vi "create data log.vi"(0 "Header String":string="This is a log file of a temperature control run being done in Physics 3600 for the bug experiment. It records the time, temperature, power, and control setting for each PID update. It does so by accumulating the data and periodically saving it.", 11 "PID exp exec in":T1) -> (4 "exists":bool=TRUE, 15 "PID exp exec out":T1)   [LabVIEW 2019]
doc: "This vi prompts the user to choose whether to create a data log. If the user so chooses, a temp parameters log file is created with the given header.\n\nPaul K Dixon\nPhysics 3600\nCSUSB Physics"
uses:
  typedefs/PID exec cluster.ctl
  typedefs/bug temp file info.ctl
  globals/Bug temp globals.vi
panel:
  out "temp log file path":path
  in  "String":string="Time (ms)\tTemp (C)\tPower\tSetpoint\tCB\tItime\tIon\tDtime\tDon\tSB\tStime\tTime in SB\tSettled\tMan Pow\tMan on"
  out "file refnum out":refnum<file>
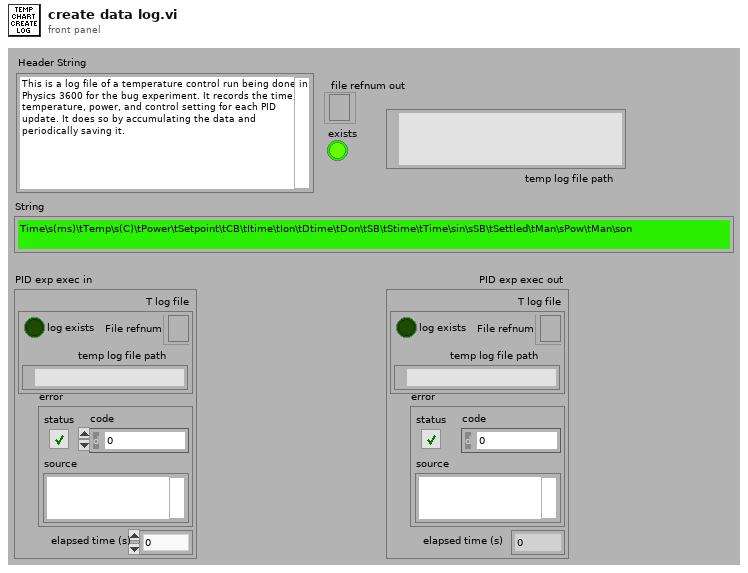
[diagram p1: front panel]
types:
  T1 = typedef "PID exec cluster.ctl" = cluster{"T log file":T2, "error":errorcluster, "elapsed time (s)":dbl}
  T2 = typedef "bug temp file info.ctl" = cluster{"log exists":bool, "File refnum":refnum<file>, "temp log file path":path}
  T3 = typedef "temp cont cluster.ctl" = cluster{"exec":T4, "T status":T6, "T params":T8, "utility":T9}
  T4 = typedef "temp exec cluster.ctl" = cluster{"T mode":T5, "exec setpoint":dbl, "reset":bool, "man power":dbl, "man":bool, "log":bool, "clear":bool}
  T5 = typedef "temp mode enum.ctl" = enum16{"Setting up", "Listening to exec", "Exit"}
  T6 = typedef "temp indicator.ctl" = cluster{"Control status":T7, "Temp":dbl, "Power":dbl, "Time in settle band":dbl, "Settled":bool, "Low":bool, "High":bool, "Setpoint":dbl, "Control":bool, "In Settle Band":bool}
  T7 = typedef "temp control status.ctl" = enum16{"In Settle Band", "In Control Band", "Below Control Band", "Above Control Band"}
  T8 = typedef "PID control parameters.ctl" = cluster{"Setpoint":dbl, "Control Bandwidth":dbl, "Integral Time":dbl, "Int\nON":bool, "Derivative Tme":dbl, "Der\nON":bool, "Settle Bandwidth":dbl, "Settle Time":dbl}
  T9 = typedef "temp cont utility.ctl" = cluster{"meas index":i32, "wait (ms)":i32, "H Vmax":dbl, "power out":dbl, "heat volt out":dbl, "heat volt in":dbl, "therm volt":dbl, "t T P hist":dbl[][], "cont hist":dbl[][]}
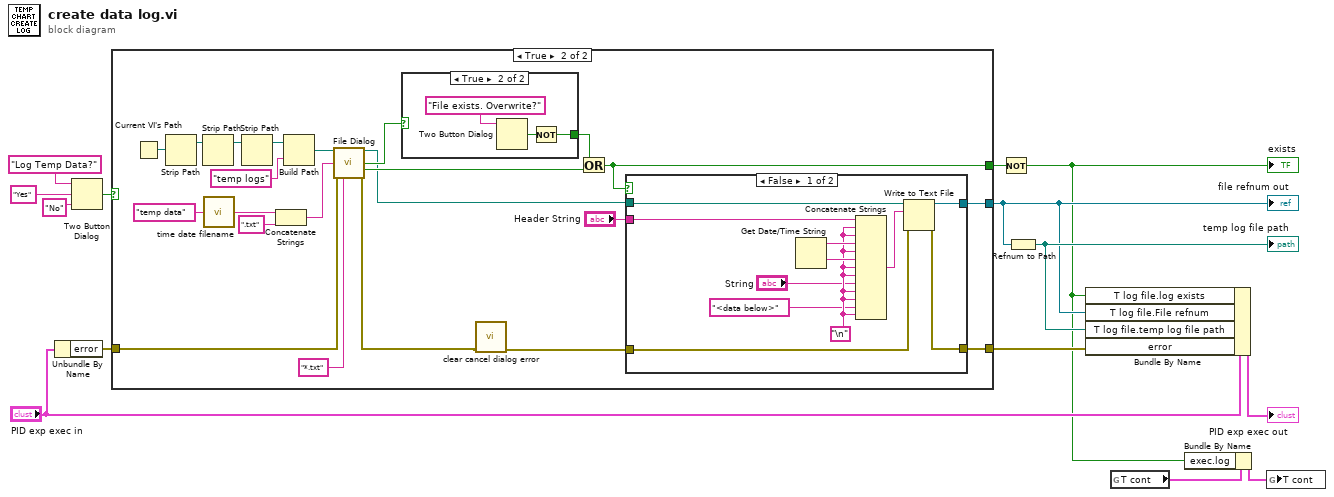
[diagram p0: block diagram]
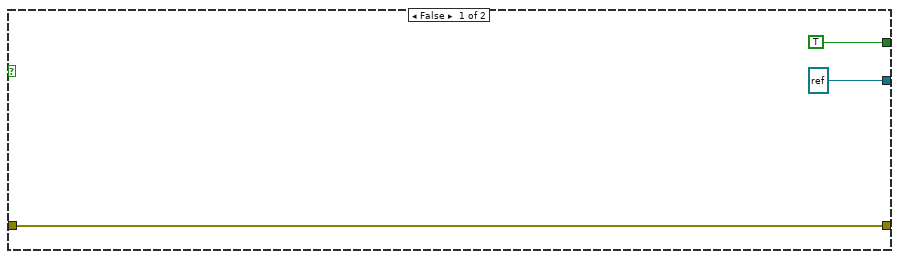
[diagram p2: hidden frame]
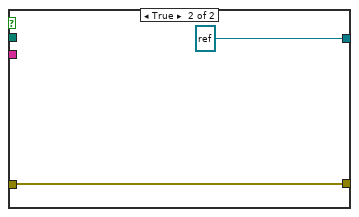
[diagram p3: hidden frame]
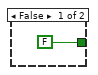
[diagram p4: hidden frame]
diagram:
  n1 = Unbundle By Name("PID exp exec in") -> ("error"=w8:errorcluster)
  n2 = Two Button Dialog(message="Log Temp Data?", 1:"No" ("F button name (\"Cancel\")"), 2:"Yes" ("T button name (\"OK\")")) -> (T button?=w10:bool)
  n3 = case shown="True" w10 {
    tunnel: [TRUE w35] -> w14
    tunnel: [w17 w33] -> w6
    tunnel: [refnum<file> refnum ("refnum out") w32] -> w4
    tunnel: w8 -> [w17 w30]
    frame False {
    }
    frame True {
      n4 = Current VI's Path() -> (path=w38:path)
      n5 = Strip Path(path=w38) -> (stripped path=w39:path)  [unwired: 1 out]
      n6 = Strip Path(path=w39) -> (stripped path=w25:path)  [unwired: 1 out]
      n7 = call "time date filename.vi"("file name in"="temp data" ("name or relative path")) -> ("time date file name out"=w20:string)  [unwired: 14 in]
      n8 = Strip Path(path=w25) -> (stripped path=w24:path)  [unwired: 1 out]
      n9 = Concatenate Strings(w20, ".txt" ("name or relative path")) -> (w18:string)
      n10 = Build Path(base path=w24, name or relative path="temp logs") -> (appended path=w22:path)
      n11 = call "File Dialog"("start path"=w22, "default name"=w18, "error in"=w30, "pattern (all files)"="*.txt") -> ("selected path"=w27:path, "exists"=w29:bool, "cancelled"=w28:bool, "error out"=w26:errorcluster)  [unwired: 8 in]
      n12 = case shown="True" w29 {
        tunnel: [FALSE ("T button?") w54] -> w37
        frame False {
        }
        frame True {
          n13 = Two Button Dialog(message="File exists. Overwrite?") -> (T button?=w55:bool)  [unwired: 2 out]
          n14 = Not(x=w55) -> (.not. x?=w54:bool)
        }
      }
      n15 = call "clear cancel dialog error.vi"("error in"=w26) -> ("error out"=w34:errorcluster)  [unwired: 14 out]
      n16 = Or(x=w37, y=w28) -> (x .or. y?=w35:bool)
      n17 = case shown="False" w35 {
        tunnel: "Header String" -> [w43 _]
        tunnel: w27 -> [w49 _]
        tunnel: w34 -> [w48 w51]
        tunnel: [w47 w51] -> w33
        tunnel: [w46 refnum<file> refnum ("refnum out")] -> w32
        frame False {
          w42 = "\n"
          n18 = Get Date/Time String() -> (date string=w45:string, time string=w44:string)  [unwired: 3 in]
          n19 = Concatenate Strings(w43, w42, w42, w45, w42, w44, w42, w42, "String", w42, w42, "<data below>", w42) -> (w50:string)
          n20 = Write to Text File(file (use dialog)=w49, text=w50, error in=w48) -> (refnum out=w46:refnum<file>, error out=w47:errorcluster)  [unwired: 2 out]
        }
        frame True {
        }
      }
    }
  }
  "file refnum out" <- w4
  n21 = Not(x=w14) -> (.not. x?=w1:bool)
  "exists" <- w1
  n22 = Refnum to Path(1:w4) -> (0:w5:path)
  "temp log file path" <- w5
  n23 = Bundle By Name(cluster="PID exp exec in", "T log file.log exists"=w1, "T log file.File refnum"=w4, "T log file.temp log file path"=w5, "error"=w6) -> (→"PID exp exec out":T1)
  n24 = global read "Bug temp globals.vi" "T cont"() -> (w3:T3)
  n25 = Bundle By Name(cluster=w3, "exec.log"=w1) -> (w2:T3)
  n26 = global write "Bug temp globals.vi" "T cont"(w2) -> ()
